vi "AgeCalculation.vi"(7 "Language":dbl(ring), 11 "CPR":string) -> (1 "Age":i32)   [LabVIEW 2013, in "main.lvlib"]
uses:
  main.lvlib
  <vilib>/Utility/miscctls.llb/LVDateTimeRec.ctl
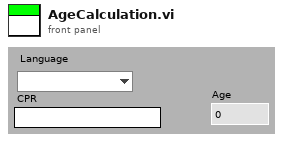
[diagram p1: front panel]
types:
  T1 = typedef "LVDateTimeRec.ctl" = cluster{"fractional second":dbl, "second":i32, "minute":i32, "hour":i32, "day of month":i32, "month":i32, "year":i32, "day of week":i32, "day of year":i32, "DST":i32}
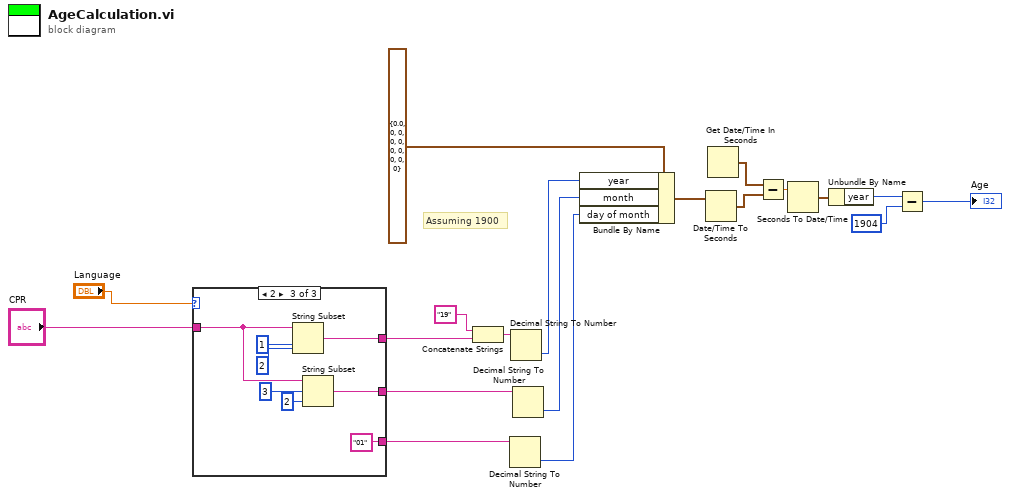
[diagram p0: block diagram]
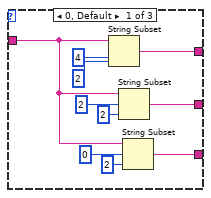
[diagram p2: hidden frame]
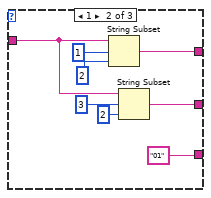
[diagram p3: hidden frame]
diagram:
  # "Assuming 1900"
  n1 = case shown="2" "Language" {
    tunnel: [w29 w37 w45] -> w15
    tunnel: [w28 "01" "01" ("CPR")] -> w10
    tunnel: [w27 w36 w44] -> w9
    tunnel: "CPR" -> [w20 w31 w39]
    frame 0, Default {
      n2 = String Subset(string=w20, offset (0)=4, length (rest)=2 ("length (rest)")) -> (substring=w29:string)
      n3 = String Subset(string=w20, offset (0)=2, length (rest)=2 ("length (rest)")) -> (substring=w27:string)
      n4 = String Subset(string=w20, offset (0)=0, length (rest)=2 ("length (rest)")) -> (substring=w28:string)
    }
    frame 1 {
      n5 = String Subset(string=w31, offset (0)=1, length (rest)=2 ("length (rest)")) -> (substring=w37:string)
      n6 = String Subset(string=w31, offset (0)=3, length (rest)=2 ("length (rest)")) -> (substring=w36:string)
    }
    frame 2 {
      n7 = String Subset(string=w39, offset (0)=1, length (rest)=2 ("length (rest)")) -> (substring=w45:string)
      n8 = String Subset(string=w39, offset (0)=3, length (rest)=2 ("length (rest)")) -> (substring=w44:string)
    }
  }
  n9 = Concatenate Strings("19" ("string"), w15) -> (w13:string)
  n10 = Decimal String To Number(string=w10) -> (number=w11:i32)  [unwired: 2 in, 1 out]
  n11 = Decimal String To Number(string=w13) -> (number=w8:i32)  [unwired: 2 in, 1 out]
  n12 = Decimal String To Number(string=w9) -> (number=w12:i32)  [unwired: 2 in, 1 out]
  n13 = Bundle By Name(cluster=T1 {"fractional second"=0.0, "second"=0, "minute"=0, "hour"=0, "day of month"=0, "month"=0, "year"=0, "day of week"=0, "day of year"=0, "DST"=0} ("date time rec"), "year"=w8, "month"=w12, "day of month"=w11) -> (w4:T1)
  n14 = Date/Time To Seconds(2:w4) -> (0:w6:timestamp)  [unwired: 1 in]
  n15 = Get Date/Time In Seconds() -> (seconds since 1Jan1904=w5:timestamp)
  n16 = Subtract(x=w5, y=w6) -> (x-y=w7:dbl)
  n17 = Seconds To Date/Time(time stamp (now)=w7) -> (date time rec=w16:T1)  [unwired: 1 in]
  n18 = Unbundle By Name(w16) -> ("year"=w17:i32)
  n19 = Subtract(x=w17, y=1904) -> (x-y=→"Age":i32)
